vi "dfd_Lattice k to Polynomial.vi"(1 "k":dbl[](array[numeric]) format="%.2f") -> (0 "poly":dbl[](array[numeric]) format="%.2f")   [LabVIEW 2017, in "NI_DigFilterLicensed.lvlib"]
uses:
  <vilib>/addons/Digital Filter Design/NI_DigFilterLicensed.lvlib
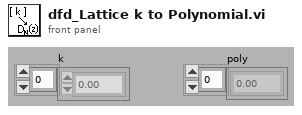
[diagram p1: front panel]
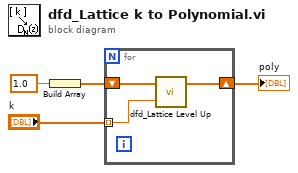
[diagram p0: block diagram]
diagram:
  n1 = Build Array(1.0 ("element")) -> (w2:dbl[])
  n2 = for {
    shift-right: [w5] -> w4
    shift-left: w2 -> [w7]
    tunnel: "k" -> [w6] mode=indexing
    n3 = call <vilib>:"dfd_Lattice Level Up.vi"("km"=w6, "Bm-1(z)"=w7) -> ("Bm(z)"=w5:dbl[])
  }
  "poly" <- w4
